vi "solar_type Set Bits.vi"(8 "Value (Binary)":string, 9 "Bit Size (32)":i32=32, 10 "Bit Offset (0)":i32, 11 "Buffered Data in":string) -> (3 "Buffered Data with Value":string)   [LabVIEW 2018]
doc: "This VI sets the length field in the <b>Data</b> string by <b>Bit Offset</b> and <b>Bit Size</b>. The total length is subtracted by the <b>Bytes to Subtract</b> parameter."
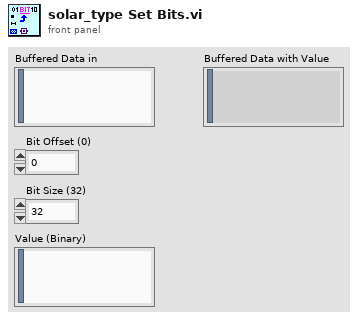
[diagram p1: front panel]
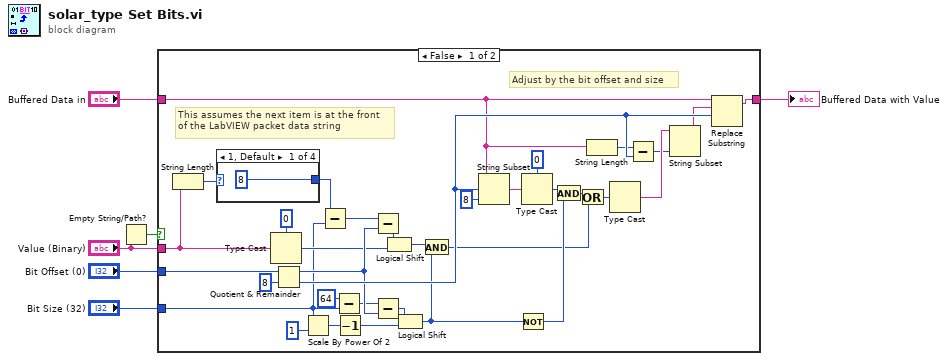
[diagram p0: block diagram]
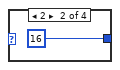
[diagram p2: hidden frame]
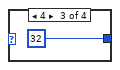
[diagram p3: hidden frame]
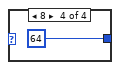
[diagram p4: hidden frame]
diagram:
  n1 = Empty String/Path?(string/path="Value (Binary)") -> (empty?=w1:bool)
  n2 = case shown="False" w1 {
    tunnel: "Buffered Data in" -> [w12 w45]
    tunnel: [w11 w45] -> w5
    tunnel: "Bit Offset (0)" -> [w10 _]
    tunnel: "Value (Binary)" -> [w9 _]
    tunnel: "Bit Size (32)" -> [w7 _]
    frame False {
      # "Adjust by the bit offset and size"
      # "This assumes the next item is at the front\nof the LabVIEW packet data string"
      n3 = String Length(string=w9) -> (length=w36:i32)
      n4 = case shown="1, Default" w36 {
        tunnel: [8 16 32 64] -> w18
        frame 1, Default {
        }
        frame 2 {
        }
        frame 4 {
        }
        frame 8 {
        }
      }
      n5 = Type Cast(type=u64 0, x=w9) -> (*(type *) &x=w37:u64)
      n6 = Quotient & Remainder(x=w10, y=8) -> (x-y*floor(x/y)=w38:i32, floor(x/y)=w39:i32)
      n7 = Scale By Power Of 2(n=w7, x=u64 1) -> (x*2^n=w25:u64)
      n8 = Subtract(x=w18, y=w7) -> (x-y=w17:i32)
      n9 = Subtract(x=64, y=w7) -> (x-y=w14:i32)
      n10 = Decrement(x=w25) -> (x-1=w26:u64)
      n11 = Subtract(x=w17, y=w38) -> (x-y=w16:i32)
      n12 = Subtract(x=w14, y=w38) -> (x-y=w13:i32)
      n13 = Logical Shift(y=w16, x=w37) -> (x << y=w31:u64)
      n14 = Logical Shift(y=w13, x=w26) -> (x << y=w32:u64)
      n15 = And(x=w31, y=w32) -> (x .and. y?=w8:u64)
      n16 = String Subset(string=w12, offset (0)=w39, length (rest)=8 ("length (rest)")) -> (substring=w23:string)
      n17 = Not(x=w32) -> (.not. x?=w28:u64)
      n18 = Type Cast(type=u64 0, x=w23) -> (*(type *) &x=w27:u64)
      n19 = And(x=w27, y=w28) -> (x .and. y?=w29:u64)
      n20 = Or(x=w29, y=w8) -> (x .or. y?=w30:u64)
      n21 = String Length(string=w12) -> (length=w20:i32)
      n22 = Type Cast(x=w30) -> (*(type *) &x=w33:string)  [unwired: 1 in]
      n23 = Subtract(x=w20, y=w39) -> (x-y=w19:i32)
      n24 = String Subset(string=w33, length (rest)=w19) -> (substring=w34:string)  [unwired: 1 in]
      n25 = Replace Substring(3:w39, 4:w34, 5:w12) -> (1:w11:string)  [unwired: 2 out]
    }
    frame True {
    }
  }
  "Buffered Data with Value" <- w5
